vi "fpga_InputOverflowOR_debug.vi"(1 "Input Lines":T1, 2 "Main Clock":u32, 3 "overflow":bool) -> (0 "Output Lines":T1)   [LabVIEW 2011]
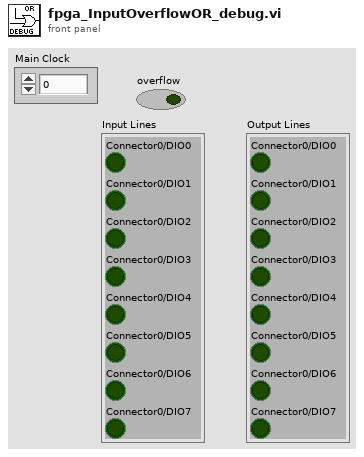
[diagram p1: front panel]
types:
  T1 = cluster{"Connector0/DIO0":bool, "Connector0/DIO1":bool, "Connector0/DIO2":bool, "Connector0/DIO3":bool, "Connector0/DIO4":bool, "Connector0/DIO5":bool, "Connector0/DIO6":bool, "Connector0/DIO7":bool}
  T2 = cluster{bool, bool, bool, bool, bool, bool, bool, bool}
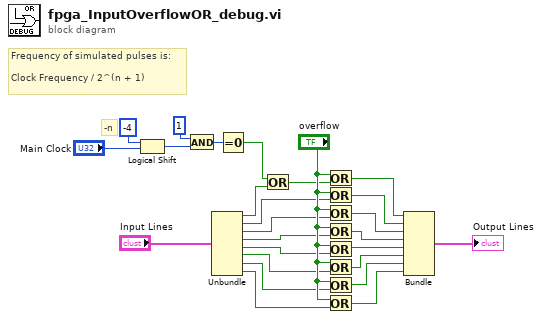
[diagram p0: block diagram]
diagram:
  # "Frequency of simulated pulses is:\n\nClock Frequency / 2^(n + 1)"
  # "-n"
  n1 = Logical Shift(y=i8 -4, x="Main Clock") -> (x << y=w4:u32)
  n2 = And(x=u32 1, y=w4) -> (x .and. y?=w7:u32)
  n3 = Unbundle("Input Lines") -> ("Connector0/DIO0"=w3:bool, "Connector0/DIO1"=w16:bool, "Connector0/DIO2"=w15:bool, "Connector0/DIO3"=w14:bool, "Connector0/DIO4"=w13:bool, "Connector0/DIO5"=w10:bool, "Connector0/DIO6"=w11:bool, "Connector0/DIO7"=w12:bool)
  n4 = Equal To 0?(x=w7) -> (x = 0?=w1:bool)
  n5 = Or(x=w1, y=w3) -> (x .or. y?=w2:bool)
  n6 = Or(x="overflow", y=w2) -> (x .or. y?=w24:bool)
  n7 = Or(x="overflow", y=w16) -> (x .or. y?=w23:bool)
  n8 = Or(x="overflow", y=w15) -> (x .or. y?=w22:bool)
  n9 = Or(x="overflow", y=w14) -> (x .or. y?=w21:bool)
  n10 = Or(x="overflow", y=w13) -> (x .or. y?=w20:bool)
  n11 = Or(x="overflow", y=w10) -> (x .or. y?=w19:bool)
  n12 = Or(x="overflow", y=w11) -> (x .or. y?=w18:bool)
  n13 = Or(x="overflow", y=w12) -> (x .or. y?=w17:bool)
  n14 = Bundle(w24, w23, w22, w21, w20, w19, w18, w17) -> (→"Output Lines":T2)  [unwired: 1 in]
